vi "Size of Variant Array.vi"(8 "error in (no error)":errorcluster, 11 "LabVIEW Array In":variant) -> (0 "error out":errorcluster, 2 "Size of Array":u32)   [LabVIEW 2010, in "i3-json.lvlib"]
uses:
  i3-json.lvlib
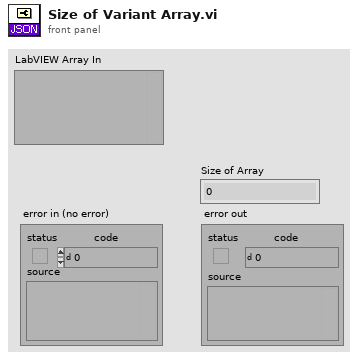
[diagram p1: front panel]
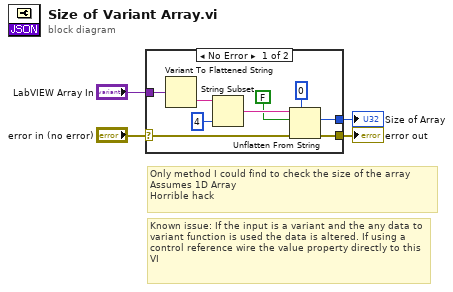
[diagram p0: block diagram]
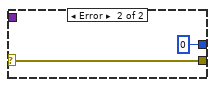
[diagram p2: hidden frame]
diagram:
  # "Known issue: If the input is a variant and the any data to variant function is used the data is altered. If using a control reference wire the value property directly to this VI"
  # "Only method I could find to check the size of the array\nAssumes 1D Array\nHorrible hack"
  n1 = case shown="No Error" "error in (no error)" {
    selector: "error in (no error)" -> [w7 w15]
    tunnel: "LabVIEW Array In" -> [w13 _]
    tunnel: [w6 w15] -> w2
    tunnel: [w5 u32 0 ("number")] -> w1
    frame No Error {
      n2 = Variant To Flattened String(Variant=w13) -> (data string=w9:string)  [unwired: 1 out]
      n3 = String Subset(string=w9, length (rest)=4 ("length (rest)")) -> (substring=w12:string)  [unwired: 1 in]
      n4 = Unflatten From String(type=u32 0 ("number"), binary string=w12, data includes array or string size? (T)=FALSE, error in (no error)=w7) -> (value=w5:u32, error out=w6:errorcluster)  [unwired: 1 in, 1 out]
    }
    frame Error {
    }
  }
  "error out" <- w2
  "Size of Array" <- w1
